vi "Run Bfr Tx - Timed Windows.vi"(7 "Process in":refnum<class "Process.lvclass">, 8 "error in (no error)":errorcluster, 11 "Tx Loop Data in":T1={"General Resources"={"Packet Name"="", "Packet ID"=0, "Local IP Address"="", "Local Port"=0, "Multicast"=FALSE, "Multicast IP Address"=0, "Header Info"=[], "Byte Order"=enum."big-endian, network order", "Channel Data Types"=[], "Duplex Packets"=refnum}, "Header Details"={"Packet Size"=0, "Protocol Revision"=0, "System Definition Version"=0, "Source Node Name"="", "Packet ID"=0, "Number of Channels"=0, "Static Header Size"=0, "Total Header Size"=0, "CustomHeaderLogic"={"CustomHeaderON"=FALSE, "CustomHeaderLogic"=""}}, "Buffer Resources"={"Data Buffer"=0, "Pointer Encoding"=enum."Direct Encoding", "Buffer Size"=0, "Buffer Size (I32)"=0, "Raw Buffer Data"=[], "Is Buffered"=FALSE, "External Buffer"=FALSE, "Prepend Header"=FALSE, "Valid Buffer"=FALSE}, "Runtime Resources"={"Connection ID"=refnum, "Transmit Option"=enum."Always", "Destination IP Address"=0, "Destination Port"=0, "Multicast IP Address"=0, "TTL"=0, "Multicast"=FALSE, "Port as Channel"=FALSE, "ExecutionConfig"={"Loop Period"=0, "RT Loop Period"=-2, "Untimed Period"=0, "Target Processor"=0, "Priority"=0, "Thread Management"=enum."Untimed (Default)"}}, "Echo Resources"={"Transmit Echo Option"=enum."PCL Reset", "Packet Count"=0.0, "Counter Increment"=0.0, "Transmit Values"=[]}, "Buffer Option Support"={"Buffer Option"=enum."Static Buffer", "Sim Option"=enum."No Simulation"}, "Channel Resources"={"Transmit Flag"=refnum, "Transmit Echo"=refnum, "Transmit Bytes"=refnum, "Port Channel"=refnum, "Buffer (External)"=refnum, "Buffer (Local)"=refnum, "Timestamp"=refnum}, "Debug Resources"={"Debug Mode"=FALSE, "Debug Log File"=refnum, "Packet Name"=""}} {"Buffer Resources"."Data Buffer" format="%016x"}) -> (3 "Tx Loop Data out":T1={"General Resources"={"Packet Name"="", "Packet ID"=0, "Local IP Address"="", "Local Port"=0, "Multicast"=FALSE, "Multicast IP Address"=0, "Header Info"=[], "Byte Order"=enum."big-endian, network order", "Channel Data Types"=[], "Duplex Packets"=refnum}, "Header Details"={"Packet Size"=0, "Protocol Revision"=0, "System Definition Version"=0, "Source Node Name"="", "Packet ID"=0, "Number of Channels"=0, "Static Header Size"=0, "Total Header Size"=0, "CustomHeaderLogic"={"CustomHeaderON"=FALSE, "CustomHeaderLogic"=""}}, "Buffer Resources"={"Data Buffer"=0, "Pointer Encoding"=enum."Direct Encoding", "Buffer Size"=0, "Buffer Size (I32)"=0, "Raw Buffer Data"=[], "Is Buffered"=FALSE, "External Buffer"=FALSE, "Prepend Header"=FALSE, "Valid Buffer"=FALSE}, "Runtime Resources"={"Connection ID"=refnum, "Transmit Option"=enum."Always", "Destination IP Address"=0, "Destination Port"=0, "Multicast IP Address"=0, "TTL"=0, "Multicast"=FALSE, "Port as Channel"=FALSE, "ExecutionConfig"={"Loop Period"=0, "RT Loop Period"=-2, "Untimed Period"=0, "Target Processor"=0, "Priority"=0, "Thread Management"=enum."Untimed (Default)"}}, "Echo Resources"={"Transmit Echo Option"=enum."PCL Reset", "Packet Count"=0.0, "Counter Increment"=0.0, "Transmit Values"=[]}, "Buffer Option Support"={"Buffer Option"=enum."Static Buffer", "Sim Option"=enum."No Simulation"}, "Channel Resources"={"Transmit Flag"=refnum, "Transmit Echo"=refnum, "Transmit Bytes"=refnum, "Port Channel"=refnum, "Buffer (External)"=refnum, "Buffer (Local)"=refnum, "Timestamp"=refnum}, "Debug Resources"={"Debug Mode"=FALSE, "Debug Log File"=refnum, "Packet Name"=""}} {"Buffer Resources"."Data Buffer" format="%016x"})   [LabVIEW 2019, in "UDP-Custom-Device Engine.lvlib"]
uses:
  UDP-Custom-Device Engine.lvlib
  <vilib>/NI/NIVS Inline Async API/_VS Inline Async API/Process/Process.lvclass
  Types/Engine - Buffered Tx Loop Data.ctl
  Types/Engine - General Resources.ctl
  <vilib>/NI VeriStand/VeriStand Data/Typedefs/Typedefs.Data Types.ctl
  Shared/Types/Shared - Duplex Settings.ctl
  Shared/Types/Shared - Header Details.ctl
  Shared/Types/Shared - Custom Header.ctl
  Types/Engine - Buffer Resources.ctl
  Shared/Types/Shared - Pointer Encoding.ctl
  Types/Engine - Tx Runtime Resources.ctl
  Shared/Types/Shared - Transmit Flag Options.ctl
  Types/Engine - Execution Config.ctl
  Shared/Types/Shared - Thread Management.ctl
  Types/Engine - Tx Echo Resources.ctl
  Shared/Types/Shared - Transmit Echo Options.ctl
  Types/Engine - Buffered Tx Buffer Option Support.ctl
  Shared/Types/Shared - Transmit Buffer Options.ctl
  Shared/Types/Shared - Transmit Sim Options.ctl
  Types/Engine - Buffered Tx Channel Refs.ctl
  <vilib>/NI/NIVS Inline Async API/_Data Access Engine/Data Access Engine/Types/Read.DVR.ctl
  <vilib>/NI/NIVS Inline Async API/_Data Access Engine/Access Type Classes/Read/Read.lvclass
  <vilib>/NI/NIVS Inline Async API/_Data Access Engine/Data Access Engine/Types/Write.DVR.ctl
  <vilib>/NI/NIVS Inline Async API/_Data Access Engine/Access Type Classes/Write/Write.lvclass
  Types/Engine - Debug Resources.ctl
  <vilib>/Platform/TimedLoop/XDataNode/timing_clust.ctl
  <vilib>/Platform/TimedLoop/XDataNode/nitl_modes.ctl
  <vilib>/Platform/TimedLoop/XDataNode/wakeup.ctl
  <vilib>/NI/NIVS Inline Async API/_Data Access Engine/Access Type Classes/Read/Read.lvclass/Read.ctl
  <vilib>/NI/NIVS Inline Async API/_Data Access Engine/Access Type Classes/Write/Write.lvclass/Write.ctl
  <vilib>/NI/NIVS Inline Async API/_VS Inline Async API/Process/Process.lvclass/Process.ctl
  <vilib>/NI VeriStand/VeriStand Data/Pointer Operations/Pointer.Write.vi
  <vilib>/NI VeriStand/VeriStand Data/Pointer Operations/Pointer.Write (String).vi
  <vilib>/NI VeriStand/VeriStand Data/Pointer Operations/Pointer.Write (1D U8).vi
  <vilib>/NI VeriStand/VeriStand Data/Pointer Operations/Pointer.Write (I32).vi
  <vilib>/NI VeriStand/VeriStand Data/Pointer Operations/Pointer.Write (U16).vi
  <vilib>/NI/NIVS Inline Async API/_Data Access Engine/Data Access Engine/Methods/Data.Processes.Execute.vi
  <vilib>/NI/NIVS Inline Async API/_Data Access Engine/Data Access Engine/Methods/Read.Data.vi
  Transmit/Run Tx - Handle Transmit Option.vi
  Run Bfr Tx - Handle Transmit Size.vi
  Transmit/Run Tx - Handle Port Tx Check.vi
  <vilib>/NI/NIVS Inline Async API/_Data Access Engine/Data Access Engine/Methods/Write.Data.vi
  <vilib>/NI VeriStand/VeriStand Data/Pointer Operations/Pointer.In-Place Read.vi
  <vilib>/NI VeriStand/VeriStand Data/Pointer Operations/Pointer.In-Place Read (1D U8).vi
  Run Bfr Tx - FIFO Entry Size.vi
  Run Bfr Tx - FIFO Payload.vi
  Run Bfr Tx - FIFO Count Packets.vi
  Run Bfr Tx - FIFO Port.vi
  <vilib>/NI/NIVS Inline Async API/_VS Inline Async API/Error Handling Process/SubVIs/Error.ConvertArray.vi
  <vilib>/NI/NIVS Inline Async API/_Data Access Engine/Access Type Classes/Read/Read.ProcessData.vi
  <vilib>/NI VeriStand/VeriStand Data/Type Conversion/Type Conversion.From Double.vi
  <vilib>/NI VeriStand/VeriStand Data/Type Conversion/Type Conversion.From Double (I32).vi
  <vilib>/NI/NIVS Inline Async API/_Data Access Engine/Access Type Classes/Write/Write.ProcessData.vi
  <vilib>/NI VeriStand/VeriStand Data/Pointer Operations/Pointer.Read.vi
  <vilib>/NI VeriStand/VeriStand Data/Pointer Operations/Pointer.Read (I32).vi
  <vilib>/NI VeriStand/VeriStand Data/Pointer Operations/Pointer.Read (U16).vi
  <vilib>/NI VeriStand/VeriStand Data/Pointer Operations/Pointer.In-Place Read (I32).vi
  <vilib>/NI VeriStand/VeriStand Data/Pointer Operations/Pointer.In-Place Read (U16).vi
  <vilib>/platform/TimedLoop/XDataNode/XDataNode.xnode
  <vilib>/Platform/TimedLoop/XDataNode/XDNodeRunTimeDep.lvlib
  <vilib>/NI VeriStand/VeriStand Data/VeriStand Data.lvlib
  Shared/UDP-Custom-Device Shared.lvlib
  <vilib>/NI/NIVS Inline Async API/_Data Access Engine/Data Access Engine/Data Access Engine.lvclass
panel:
  out "dataBuffer":u64 format="%016x"
  out "Tx Packet":string
  # "BUFFERED TRANSMIT\n- TIMED\n- WINDOWS ONLY"
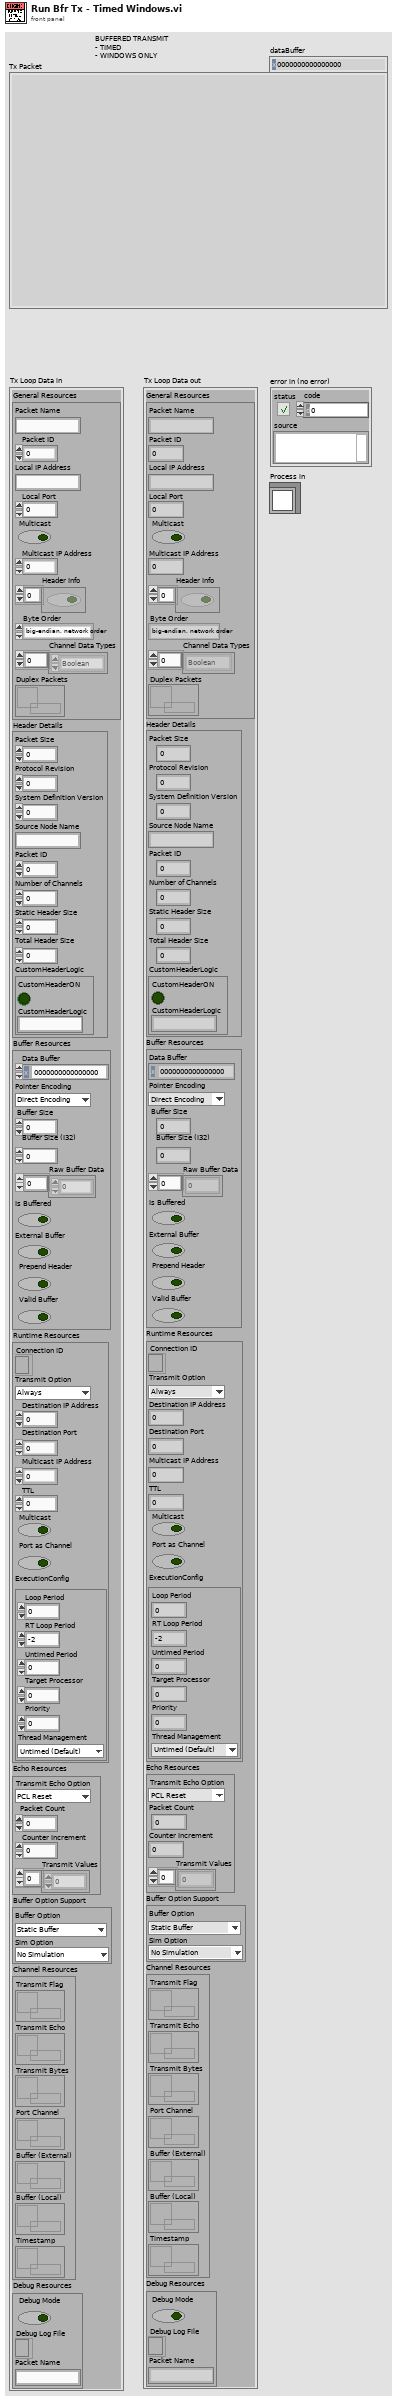
[diagram p1: front panel]
types:
  T1 = typedef "UDP-Custom-Device Engine.lvlib/Engine - Buffered Tx Loop Data.ctl" = cluster{"General Resources":T2, "Header Details":T4, "Buffer Resources":T6, "Runtime Resources":T8, "Echo Resources":T12, "Buffer Option Support":T14, "Channel Resources":T17, "Debug Resources":T20}
  T2 = typedef "UDP-Custom-Device Engine.lvlib/Engine - General Resources.ctl" = cluster{"Packet Name":string, "Packet ID":i32, "Local IP Address":string, "Local Port":i32, "Multicast":bool, "Multicast IP Address":u32, "Header Info":bool[], "Byte Order":enum16{"big-endian, network order", "native, host order", "little-endian"}, "Channel Data Types":T3[], "Duplex Packets":refnum<data-value>}
  T3 = typedef "VeriStand Data.lvlib/Typedefs.Data Types.ctl" = enum16{"Boolean", "Single", "Double", "I8", "I16", "I32", "I64", "U8", "U16", "U32", "U64"}
  T4 = typedef "UDP-Custom-Device Shared.lvlib/Shared - Header Details.ctl" = cluster{"Packet Size":u16, "Protocol Revision":u8, "System Definition Version":u64, "Source Node Name":string, "Packet ID":u32, "Number of Channels":u32, "Static Header Size":u16, "Total Header Size":u16, "CustomHeaderLogic":T5}
  T5 = typedef "UDP-Custom-Device Shared.lvlib/Shared - Custom Header.ctl" = cluster{"CustomHeaderON":bool, "CustomHeaderLogic":string}
  T6 = typedef "UDP-Custom-Device Engine.lvlib/Engine - Buffer Resources.ctl" = cluster{"Data Buffer":u64, "Pointer Encoding":T7, "Buffer Size":u64, "Buffer Size (I32)":i32, "Raw Buffer Data":u8[], "Is Buffered":bool, "External Buffer":bool, "Prepend Header":bool, "Valid Buffer":bool}
  T7 = typedef "UDP-Custom-Device Shared.lvlib/Shared - Pointer Encoding.ctl" = enum16{"Direct Encoding", "Conversion Encoding"}
  T8 = typedef "UDP-Custom-Device Engine.lvlib/Engine - Tx Runtime Resources.ctl" = cluster{"Connection ID":refnum<k16>, "Transmit Option":T9, "Destination IP Address":u32, "Destination Port":u16, "Multicast IP Address":u32, "TTL":u16, "Multicast":bool, "Port as Channel":bool, "ExecutionConfig":T10}
  T9 = typedef "UDP-Custom-Device Shared.lvlib/Shared - Transmit Flag Options.ctl" = enum16{"Always", "One-Shot", "Toggle"}
  T10 = typedef "UDP-Custom-Device Engine.lvlib/Engine - Execution Config.ctl" = cluster{"Loop Period":i64, "RT Loop Period":i64, "Untimed Period":u32, "Target Processor":i32, "Priority":i32, "Thread Management":T11}
  T11 = typedef "UDP-Custom-Device Shared.lvlib/Shared - Thread Management.ctl" = enum16{"Untimed (Default)", "Timed (High Priority)"}
  T12 = typedef "UDP-Custom-Device Engine.lvlib/Engine - Tx Echo Resources.ctl" = cluster{"Transmit Echo Option":T13, "Packet Count":dbl, "Counter Increment":dbl, "Transmit Values":dbl[]}
  T13 = typedef "UDP-Custom-Device Shared.lvlib/Shared - Transmit Echo Options.ctl" = enum16{"PCL Reset", "Counter", "Mirror"}
  T14 = typedef "UDP-Custom-Device Engine.lvlib/Engine - Buffered Tx Buffer Option Support.ctl" = cluster{"Buffer Option":T15, "Sim Option":T16}
  T15 = typedef "UDP-Custom-Device Shared.lvlib/Shared - Transmit Buffer Options.ctl" = enum16{"Static Buffer", "FIFO Buffer", "FIFO Buffer + Port"}
  T16 = typedef "UDP-Custom-Device Shared.lvlib/Shared - Transmit Sim Options.ctl" = enum16{"No Simulation", "Counter", "Full Buffer", "FIFO Test", "FIFO + Port Test"}
  T17 = typedef "UDP-Custom-Device Engine.lvlib/Engine - Buffered Tx Channel Refs.ctl" = cluster{"Transmit Flag":T18, "Transmit Echo":T19, "Transmit Bytes":T18, "Port Channel":T18, "Buffer (External)":T18, "Buffer (Local)":T19, "Timestamp":T18}
  T18 = typedef "Data Access Engine.lvlib/Data Access Engine.lvclass/Read.DVR.ctl" = refnum<data-value>
  T19 = typedef "Data Access Engine.lvlib/Data Access Engine.lvclass/Write.DVR.ctl" = refnum<data-value>
  T20 = typedef "UDP-Custom-Device Engine.lvlib/Engine - Debug Resources.ctl" = cluster{"Debug Mode":bool, "Debug Log File":refnum<file>, "Packet Name":string}
  T21 = typedef "XDNodeRunTimeDep.lvlib/timing_clust.ctl" = cluster{"Expected End [f-1]":u64, "Actual End [f-1]":u64, "Finished Late? [f-1]":bool, "Expected End [i-1]":u64, "Actual End [i-1]":u64, "Finished Late? [i-1]":bool, "Expected Start [i]":u64, "Actual Start [i]":u64, "Expected Start [f]":u64, "Actual Start [f]":u64, "Source Name":string, "Structure Name":string, "Period":i64, "Deadline":i64, "Offset":i64, "Start":i64, "Priority":i32, "Timeout":i32, "Mode":T22, "Wakeup Reason":T23, "Error":errorcluster, "Source Type":string, "Secondary Source Type":string, "Global End Time":u64, "Global Start Time":u64, "Frame Duration":u64, "Iteration Duration":u64, "Assigned CPU":i32, "I/O Scan Engine Mode":u32}
  T22 = typedef "XDNodeRunTimeDep.lvlib/nitl_modes.ctl" = enum32{"No Change", "Process missed periods, maintain original phase", "Discard missed periods, maintain original phase", "Process missed periods, ignore original phase", "Discard missed periods, ignore original phase"}
  T23 = typedef "XDNodeRunTimeDep.lvlib/wakeup.ctl" = enum32{"Normal", "Aborted", "Asynchronous wakeup", "Timing source error", "Timed loop error", "Timeout"}
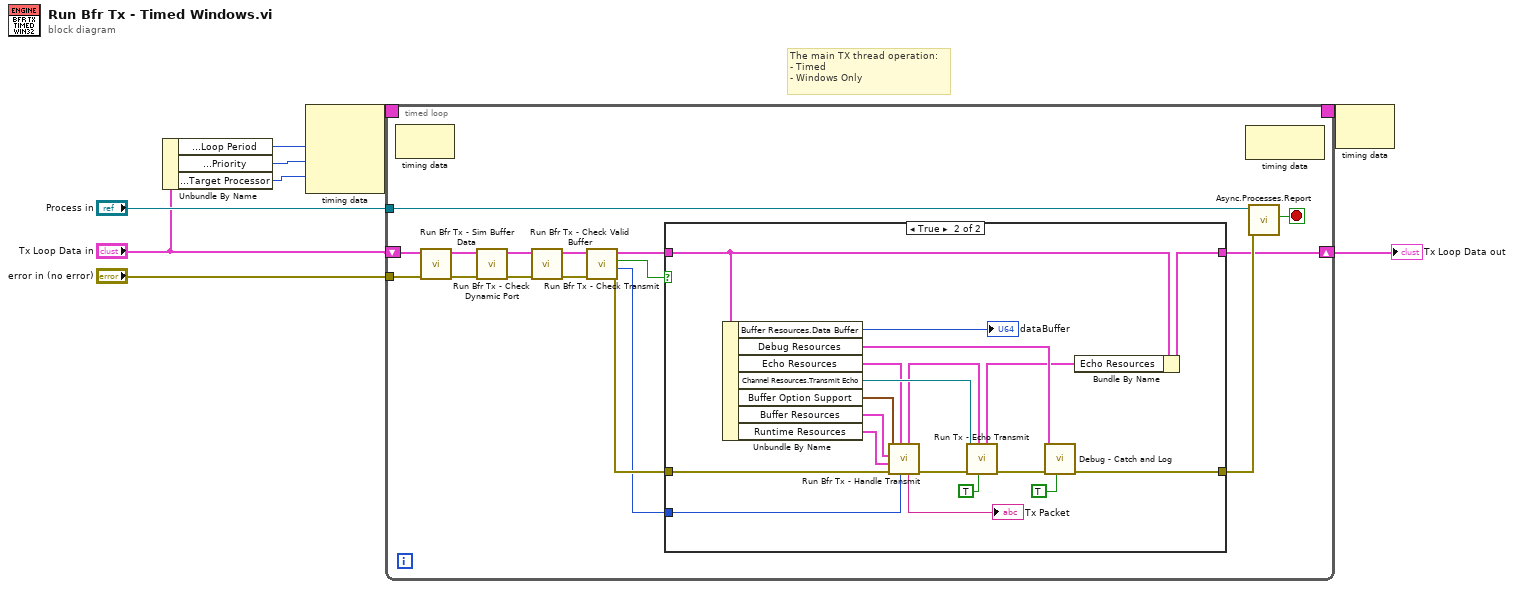
[diagram p0: block diagram]
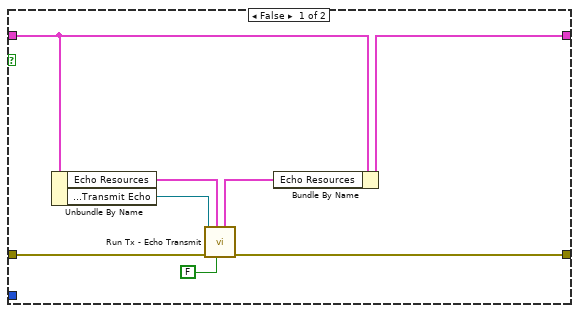
[diagram p2: hidden frame]
diagram:
  # "The main TX thread operation:\n- Timed\n- Windows Only"
  n1 = Unbundle By Name("Tx Loop Data in") -> ("Runtime Resources.ExecutionConfig.Loop Period"=w7:i64, "Runtime Resources.ExecutionConfig.Priority"=w6:i32, "Runtime Resources.ExecutionConfig.Target Processor"=w5:i32)
  n2 = node-c288(w7, w6, w5) -> (w9:T21)  [unwired: 1 in]
  n3 = timed-loop {
    tunnel: "error in (no error)" -> [w21]
    tunnel: "Process in" -> [w25]
    shift-right: [w20] -> w1
    shift-left: "Tx Loop Data in" -> [w22]
    timing: w9 -> [_]
    timing-out: [_] -> w8
    stop <- w24 stop-if-true
    n4 = node-c288() -> ()  [unwired: 1 in, 1 out]
    n5 = call "Run Bfr Tx - Sim Buffer Data.vi"("error in (no error)"=w21, "Tx Loop Data in"=w22) -> ("error out"=w11:errorcluster, "Tx Loop Data out"=w13:T1)  [unwired: 8 in]
    n6 = call "Run Bfr Tx - Check Dynamic Port.vi"("error in (no error)"=w11, "Tx Loop Data in"=w13) -> ("error out"=w10:errorcluster, "Tx Loop Data out"=w12:T1)  [unwired: 8 in]
    n7 = call "Run Bfr Tx - Check Valid Buffer.vi"("error in (no error)"=w10, "Tx Loop Data in"=w12) -> ("error out"=w14:errorcluster, "Tx Loop Data out"=w15:T1)  [unwired: 8 in]
    n8 = call "Run Bfr Tx - Check Transmit.vi"("error in (no error)"=w14, "Tx Loop Data in"=w15) -> ("error out"=w19:errorcluster, "Bytes to Transmit"=w16:i32, "Transmit?"=w18:bool, "Tx Loop Data out"=w17:T1)  [unwired: 6 in]
    n9 = case shown="True" w18 {
      tunnel: [w28 w49] -> w23
      tunnel: [w31 w51] -> w20
      tunnel: w19 -> [w34 w46]
      tunnel: w17 -> [w32 w52]
      tunnel: w16 -> [_ w44]
      frame False {
        n10 = Unbundle By Name(w32) -> ("Echo Resources"=w30:T12, "Channel Resources.Transmit Echo"=w35:T19)
        n11 = call "Run Tx - Echo Transmit.vi"("Transmitted?"=FALSE, "Echo Resources in"=w30, "error in (no error)"=w34, "Ref"=w35) -> ("error out"=w28:errorcluster, "Echo Resources out"=w29:T12)  [unwired: 6 in]
        n12 = Bundle By Name(cluster=w32, "Echo Resources"=w29) -> (w31:T1)
      }
      frame True {
        n13 = Unbundle By Name(w52) -> ("Buffer Resources.Data Buffer"=→"dataBuffer":u64, "Debug Resources"=w48:T20, "Echo Resources"=w40:T12, "Channel Resources.Transmit Echo"=w54:T19, "Buffer Option Support"=w41:T14, "Buffer Resources"=w42:T6, "Runtime Resources"=w43:T8)
        n14 = call "Run Bfr Tx - Handle Transmit.vi"("Bytes to Transmit"=w44, "Echo Resources in"=w40, "error in (no error)"=w46, "Runtime Resources"=w43, "Buffer Resources"=w42, "Buffer Option Support in"=w41) -> ("error out"=w45:errorcluster, "Tx Packet"=→"Tx Packet":string, "Echo Resources out"=w39:T12)  [unwired: 3 in]
        n15 = call "Run Tx - Echo Transmit.vi"("Transmitted?"=TRUE, "Echo Resources in"=w39, "error in (no error)"=w45, "Ref"=w54) -> ("error out"=w38:errorcluster, "Echo Resources out"=w47:T12)  [unwired: 6 in]
        n16 = call "Debug - Catch and Log.vi"("Clear Error?"=TRUE, "error in (no error)"=w38, "Debug Resources"=w48) -> ("error out"=w49:errorcluster)  [unwired: 8 in]
        n17 = Bundle By Name(cluster=w52, "Echo Resources"=w47) -> (w51:T1)
      }
    }
    n18 = node-c288() -> ()  [unwired: 1 in, 1 out]
    n19 = call <vilib>:"Async.Processes.Report.vi"("Error"=w23, "Process in"=w25) -> ("Stop"=w24:bool)  [unwired: 8 in, 1 out]
  }
  "Tx Loop Data out" <- w1
  n20 = node-c288(w8) -> ()  [unwired: 1 out]
